vi "Set baud rate.vi"(10 "baud rate":refnum<vi>, 11 "BD Protocol 4.0 in":refnum<class "BD Protocol 4.0.lvclass">) -> (3 "BD Protocol 4.0 out":refnum<class "BD Protocol 4.0.lvclass">)   [LabVIEW 2016, in "BD Protocol 4.0.lvlib" / "BD Protocol 4.0.lvclass"]
uses:
  BD Protocol 4.0.lvclass
  BD Protocol 4.0.lvclass/BD Protocol 4.0.ctl
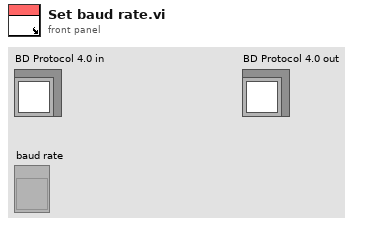
[diagram p1: front panel]
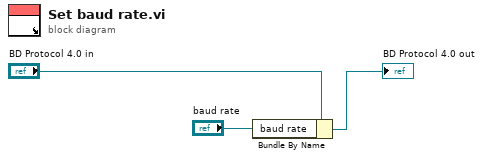
[diagram p0: block diagram]
diagram:
  n1 = Bundle By Name(cluster="BD Protocol 4.0 in", "baud rate"="baud rate") -> (→"BD Protocol 4.0 out":refnum<class "BD Protocol 4.0.lvclass">)
